vi "evaluate_timeout.vi"(7 "reset?":bool, 11 "timeout (ms)":i32) -> (2 "elapsed":bool, 3 "remaining timeout (ms)":i32)   [LabVIEW 2013, in "Connection_GOSPL.lvlib" / "Connection.lvclass"]
uses:
  Connection.lvclass
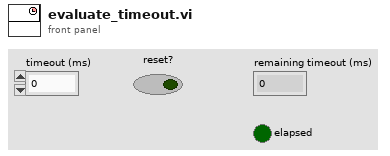
[diagram p1: front panel]
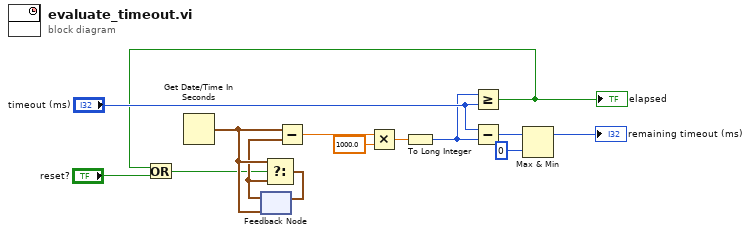
[diagram p0: block diagram]
diagram:
  n1 = Get Date/Time In Seconds() -> (seconds since 1Jan1904=w9:timestamp)
  n2 = feedback #1(w9) -> (w4:timestamp)
  n3 = Subtract(x=w9, y=w4) -> (x-y=w12:dbl)
  n4 = Multiply(x=w12, y=1000.0) -> (x*y=w11:dbl)
  n5 = To Long Integer(number=w11) -> (32bit integer=w10:i32)
  n6 = Greater Or Equal?(x=w10, y="timeout (ms)") -> (x >= y?=w1:bool)
  "elapsed" <- w1
  n7 = Or(x=w1, y="reset?") -> (x .or. y?=w3:bool)
  n8 = Select(t=w9, s=w3, f=w4) -> (s? t:f=w8:timestamp)
  n9 = feedback-in #1(w8) -> ()
  n10 = Subtract(x="timeout (ms)", y=w10) -> (x-y=w7:i32)
  n11 = Max & Min(x=w7, y=0 ("lower limit")) -> (max(x,y)=→"remaining timeout (ms)":i32)  [unwired: 1 out]
